vi "LCB Read Last Dev Err.vi"(8 "error in (no error)":errorcluster caption="Fehler (Eingang, kein Fehler)", 11 "Device Handle":i64) -> (0 "error out":errorcluster caption="Fehler (Ausgang)", 3 "Last Device Error":u32)   [LabVIEW 2021, in "labbCAN_Bus_API.lvlib"]
doc: "LCB_Func long __stdcall LCB_ReadLastDevErr(dev_hdl hDev,\n unsigned long *pDevErr);"
uses:
  labbCAN_Bus_API.lvlib
  labbCAN_Bus_API.dll
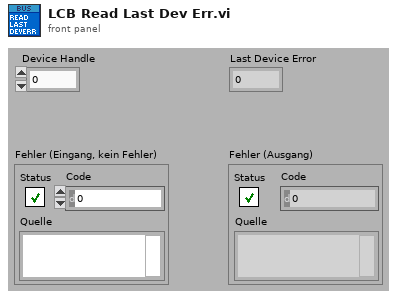
[diagram p1: front panel]
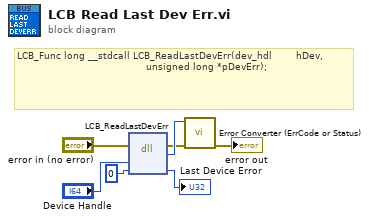
[diagram p0: block diagram]
diagram:
  # "LCB_Func long __stdcall LCB_ReadLastDevErr(dev_hdl        hDev,\n                                           unsigned long *pDevErr);"
  n1 = dll-call lib="C:/Users/olaja/AppData/Local/CETONI_SDK/labbCAN_Bus_API.*" fn="LCB_ReadLastDevErr"(error in="error in (no error)", "hDev"="Device Handle", "pDevErr"=u32 0) -> (error out=w2:errorcluster, "Rückgabetyp"=w3:i32, "pDevErr"=→"Last Device Error":u32)  [unwired: 3 in, 1 out]
  n2 = call "Error Converter (ErrCode or Status).vi"("error in (no error)"=w2, "error code"=w3) -> ("error out"=→"error out":errorcluster)  [unwired: 9 in]
